vi "Write_Data.vi"(8 "error in (no error)":errorcluster caption="entrée d'erreur (pas d'erreur)", 10 "Data_To_Write":string, 11 "Class Instrument Process en entrée":refnum<class "Class Instrument Process.lvclass">) -> (0 "error out":errorcluster caption="sortie d'erreur", 3 "Class Instrument Process en sortie":refnum<class "Class Instrument Process.lvclass">)   [LabVIEW 2020, in "Library Instrument & Equipement.lvlib" / "Library Instruments.lvlib" / "Class Instrument Process.lvclass"]
uses:
  Class Instrument Process.lvclass
  Commun VI/TypeDef/Commande Process/Commande Data Process.ctl
  JSON API/JSON Value/Set from JSON string.vi
  JSON API/JSON Value/JSON Value.lvclass
  Class Instrument Process.lvclass/Class Instrument Process.ctl
  JSON API/Variant JSON/Variant JSON.lvlib
  JSON API/Get Polymorphic/JSON GetSet.lvlib
  Commun VI/Library Commun.lvlib
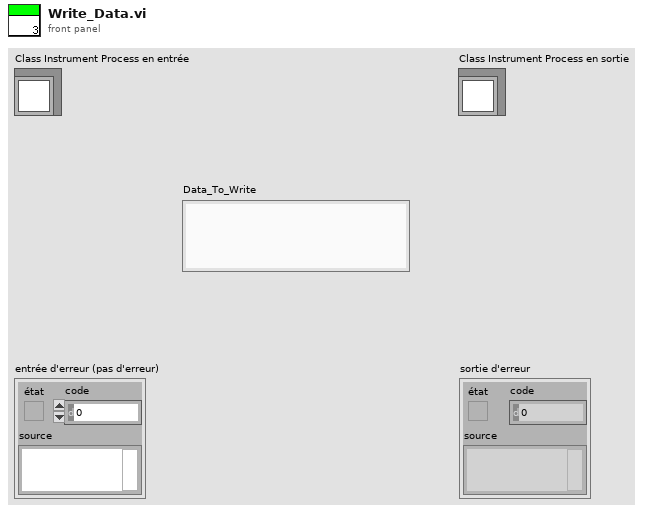
[diagram p1: front panel]
types:
  T1 = typedef "Library Commun.lvlib/Commande Data Process.ctl" = cluster{"Function":enum16{"Run", "Kill"}}
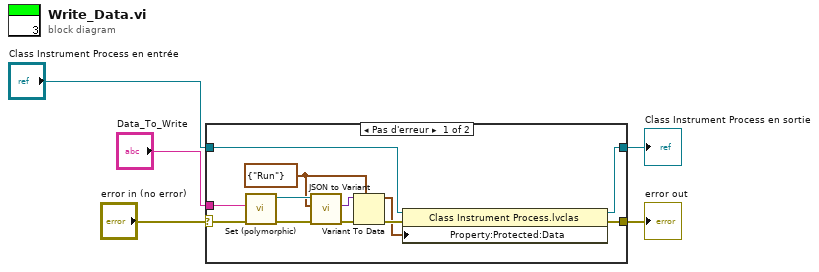
[diagram p0: block diagram]
diagram:
  n1 = case shown="Pas d'erreur" "error in (no error)" {
    selector: "error in (no error)" -> [w9 w19]
    tunnel: [w16 w19] -> w2
    tunnel: [w15 w18] -> w3
    tunnel: "Class Instrument Process en entrée" -> [w17 w18]
    tunnel: "Data_To_Write" -> [w10 _]
    frame No Error {
      w7 = T1 {"Function"=enum."Run"} ("Parameter")
      n2 = call-poly "Set (polymorphic).vi"("error in (no error)"=w9, "JSON stream"=w10) -> ("error out"=w13:errorcluster, "JSON Value out"=w11:refnum<class "JSON Value.lvclass">)  [unwired: 7 in, 1 out]
      n3 = call "JSON to Variant.vi"("error in (no error)"=w13, "Variant (Data Type)"=w7, "JSON Value"=w11) -> ("error out"=w12:errorcluster, "Variant out"=w14:variant)  [unwired: 7 in]
      n4 = Variant To Data(error in=w12, type=w7, Variant=w14) -> (data=w6:T1, error out=w8:errorcluster)
      n5 = property class="Class Instrument Process.lvclas"(reference=w17, error in=w8, "Property:Protected:Data"=w6) -> (reference out=w15:refnum<class "Class Instrument Process.lvclass">, error out=w16:errorcluster)
    }
    frame Error {
    }
  }
  "error out" <- w2
  "Class Instrument Process en sortie" <- w3
